vi "Parse Headers-Body (old).vi"(8 "error in":errorcluster, 11 "Header-Body Data":T1) -> (0 "error out":errorcluster, 3 "HTTP Status":T2)   [LabVIEW 2020, in "InfluxDB v2 Client.lvlib"]
doc: "Parses headers and body into the components:\n1) Code\n2) Status\n3) Desciption"
uses:
  InfluxDB v2 Client.lvlib
  HTTP Status.ctl
  Header-Body Data.ctl
  <vilib>/regexp/Match Regular Expression.xnode
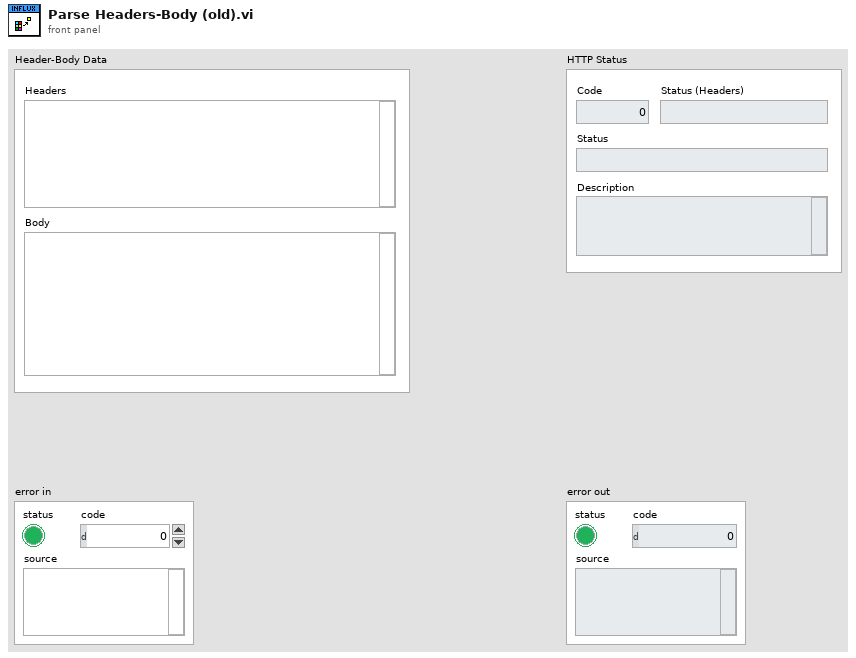
[diagram p1: front panel]
types:
  T1 = typedef "InfluxDB v2 Client.lvlib/Header-Body Data.ctl" = cluster{"Headers":string, "Body":string}
  T2 = typedef "InfluxDB v2 Client.lvlib/HTTP Status.ctl" = cluster{"Code":i32, "Status":string, "Description":string, "Status (Headers)":string}
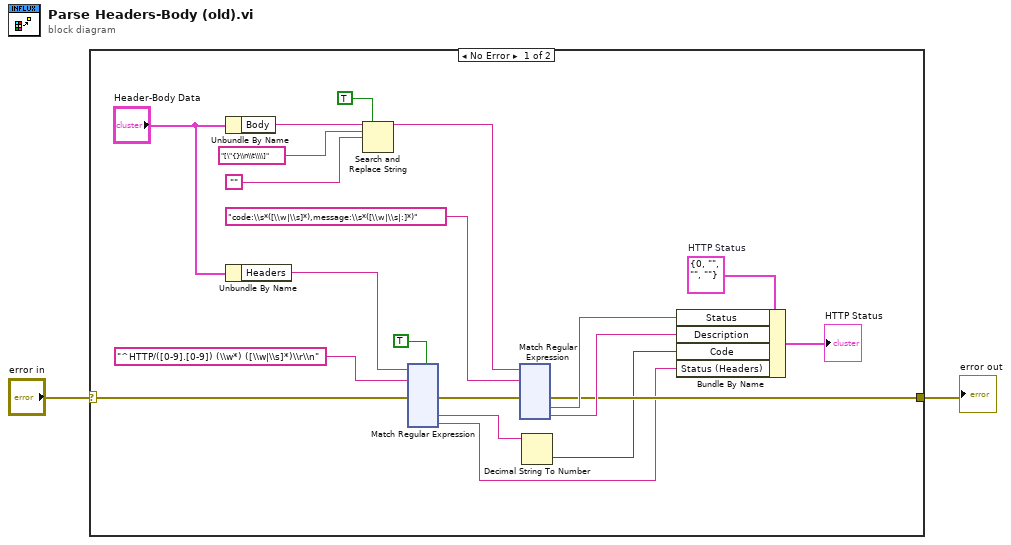
[diagram p0: block diagram]
diagram:
  n1 = case shown="No Error" "error in" {
    selector: "error in" -> [w19 w258]
    tunnel: [w5 w258] -> w1
    frame No Error {
      w10 = T2 {"Code"=0, "Status"="", "Description"="", "Status (Headers)"=""}  # HTTP Status
      n2 = Unbundle By Name("Header-Body Data") -> ("Body"=w13:string)
      n3 = Unbundle By Name("Header-Body Data") -> ("Headers"=w20:string)
      n4 = Search and Replace String(replace all?=TRUE ("replace all? (F)"), input string=w13, search string="[\"{}\\n\\t\\\\]", replace string="") -> (result string=w12:string)  [unwired: 4 in, 3 out]
      n5 = xnode "Match Regular Expression"("input string"=w20, "regular expression"="^HTTP/([0-9].[0-9]) (\\w*) ([\\w|\\s]*)\\r\\n", "error in"=w19, "multiline? (F)"=TRUE) -> ("error out"=w6:errorcluster, "submatch 2"=w18:string, "submatch 3"=w3:string)  [unwired: 2 in, 5 out]
      n6 = xnode "Match Regular Expression"("input string"=w12, "regular expression"="code:\\s*([\\w|\\s]*),message:\\s*([\\w|\\s|:]*)", "error in"=w6) -> ("error out"=w5:errorcluster, "submatch 1"=w9:string, "submatch 2"=w8:string)  [unwired: 3 in, 4 out]
      n7 = Decimal String To Number(string=w18) -> (number=w4:i32)  [unwired: 2 in, 1 out]
      n8 = Bundle By Name(cluster=w10, "Status"=w9, "Description"=w8, "Code"=w4, "Status (Headers)"=w3) -> (→"HTTP Status":T2)
    }
    frame Error {
    }
  }
  "error out" <- w1
